vi "Main.vi"() -> ()   [LabVIEW 2017, in "Vibratome.lvlib"]
uses:
  Vibratome.lvlib
  Controls/Down.ctl
  Controls/Up.ctl
  Drivers/ASI/Public/Utility/Axis Name.ctl
  Support VIs/Message Queue/Enqueue Message (Single).vi
  Support VIs/Message Queue/Enqueue Message (Multiple).vi
  Support VIs/Stop Event/Stop Event.lvlib
  Support VIs/Message Queue/Message Queue.lvlib
  Piezo Controller/Piezo Controller.lvlib
  Stage/Stage.lvlib
  Drivers/ASI/ASI TG-1000.lvlib
panel:
  in  "Specimen X":cluster{"X-":T1, "X+":T2}
  in  "Set X Pos":T3
  in  "Abort":bool
  in  "Run":bool
  in  "Specimen Z":cluster{"Z-":T1, "Z+":T2}
  in  "Blade":cluster{"F-":T1, "F+":T2}
  in  "Oscillator Settings":cluster{"Amplitude":dbl, "Frequency":dbl}={"Amplitude"=5.0, "Frequency"=40.0} {"Frequency" format="%.0f Hz"; "Amplitude" format="%.0f V"}
  in  "Speed":dbl min=0.0 step=0.1 format="%.1f mm/s"
  in  "Thickness":dbl=50.0 min=0.0 max=10000.0 step=1.0 format="%.0f um"
  # "Blade"
  # "Specimen"
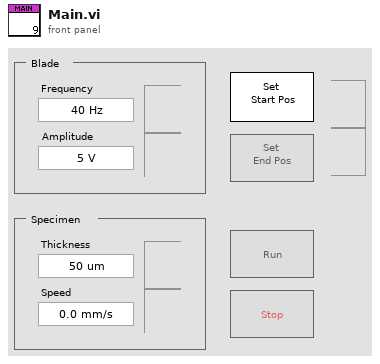
[diagram p1: front panel]
types:
  T1 = typedef "Vibratome.lvlib/Down.ctl" = bool
  T2 = typedef "Vibratome.lvlib/Up.ctl" = bool
  T3 = cluster{"Set Start Pos":bool, "Set End Pos":bool}
  T4 = typedef "Vibratome.lvlib/Message Queues.ctl" = cluster{"UI Message":refnum<queue>, "Piezo Message":refnum<queue>, "Stage Message":refnum<queue>}
  T5 = typedef "Drivers.lvlib/ASI TG-1000.lvlib/Axis Name.ctl" = enum8{"undefined", "A", "B", "C", "D", "E", "F", "G", "H", "I", "J", "K", "L", "M", "N", "O", "P", "Q", "R", "S", "T", "U", "V", "W", "X", "Y", "Z"}
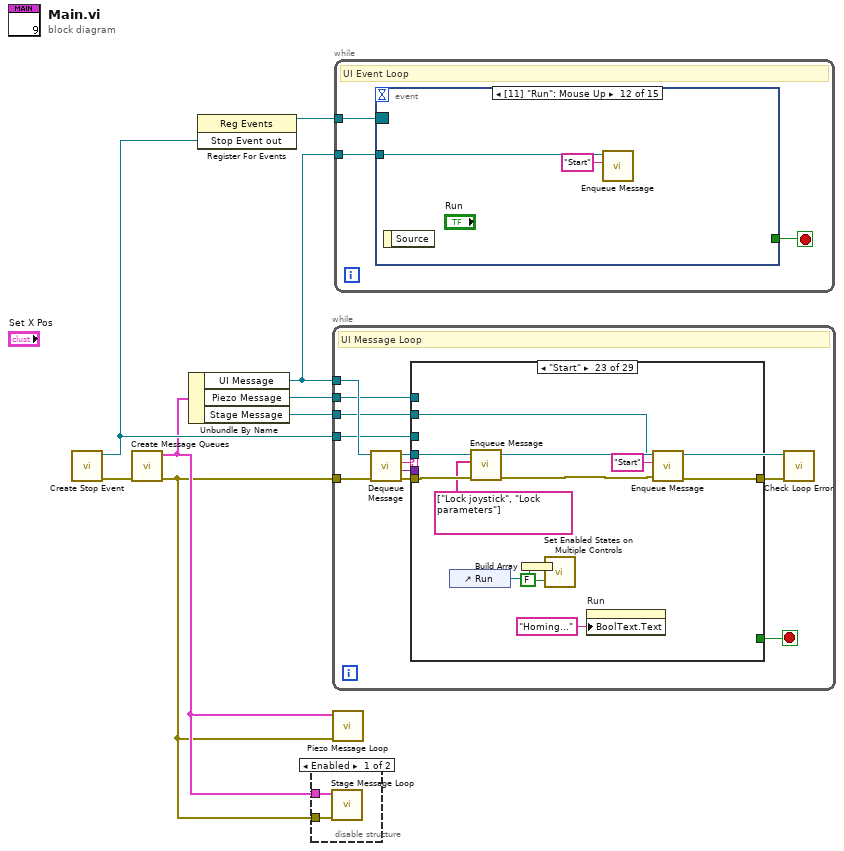
[diagram p0: block diagram]
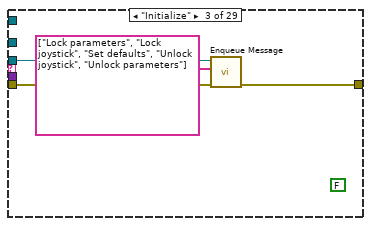
[diagram p5: hidden frame]
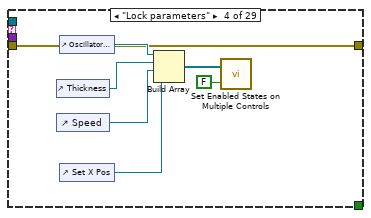
[diagram p6: hidden frame]
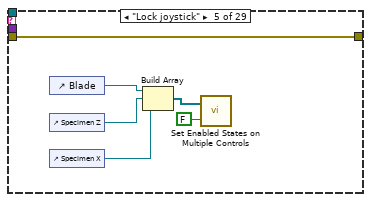
[diagram p7: hidden frame]
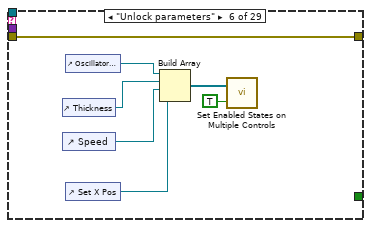
[diagram p8: hidden frame]
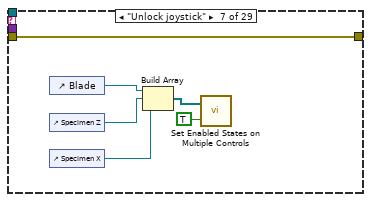
[diagram p9: hidden frame]
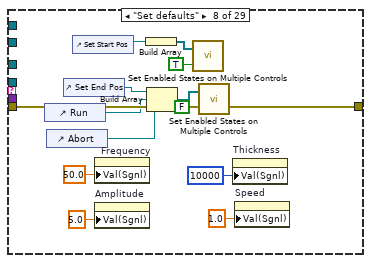
[diagram p10: hidden frame]
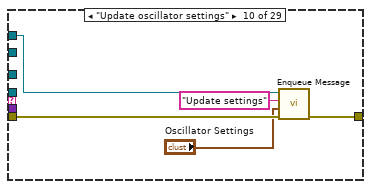
[diagram p12: hidden frame]
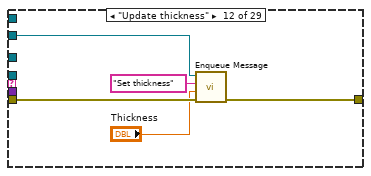
[diagram p14: hidden frame]
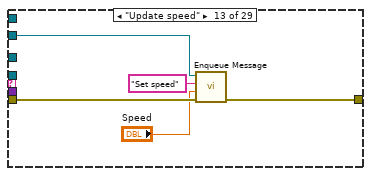
[diagram p15: hidden frame]
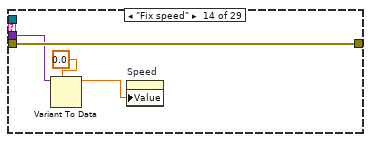
[diagram p16: hidden frame]
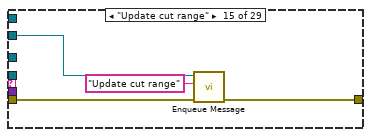
[diagram p17: hidden frame]
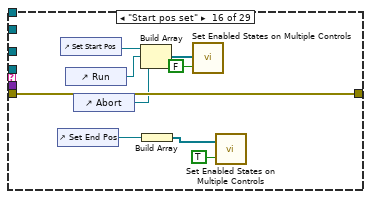
[diagram p18: hidden frame]
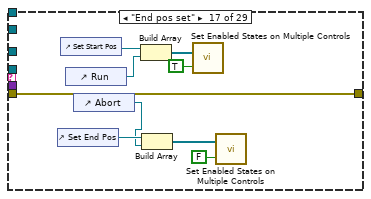
[diagram p19: hidden frame]
diagram:
  n1 = call "Create Stop Event.vi"() -> ("error out"=w8:errorcluster, "Stop Event out"=w3:refnum<user-event>)  [unwired: 10 in]
  n2 = call "Create Message Queues.vi"("error in (no error)"=w8) -> ("error out"=w1:errorcluster, "Message Queues"=w2:T4)  [unwired: 9 in]
  n3 = Unbundle By Name(w2) -> ("UI Message"=w6:refnum<queue>, "Piezo Message"=w5:refnum<queue>, "Stage Message"=w4:refnum<queue>)
  n4 = register-events(w3) -> (reference out=w7:refnum<event-registration>)  [unwired: 2 in, 1 out]
  n5 = disable-structure shown="Enabled" {
    disable-tunnel: w2 -> [w10 _]
    disable-tunnel: w1 -> [w9 _]
    frame Enabled {
      n6 = call "Stage Message Loop.vi"("error in (no error)"=w9, "Message Queues"=w10) -> ()  [unwired: 9 in, 1 out]
    }
    frame Disabled {
    }
  }
  n7 = while {
    tunnel: w6 -> [w21]
    tunnel: w1 -> [w20]
    tunnel: w5 -> [w13]
    tunnel: w4 -> [w12]
    tunnel: w3 -> [w14]
    stop <- w15 stop-if-true
    # "UI Message Loop"
    n8 = call "Dequeue Message.vi"("error in (no error)"=w20, "Message Queue in"=w21) -> ("error out"=w18:errorcluster, "Data"=w11:variant, "State"=w19:string, "Message Queue out"=w17:refnum<queue>)  [unwired: 6 in]
    n9 = case shown="\"Start\"" w19 {
      tunnel: w17 -> [_ _ w27 _ _ _ _ _ _ _ _ _ _ _ _ _ _ _ _ _ _ _ w155 _ _ w184 _ _ _]
      tunnel: w18 -> [w22 w23 w26 w28 w35 w41 w48 w62 w67 w72 w73 w78 w83 w87 w91 w100 w109 w110 w122 w134 w146 w147 w156 w160 w176 w180 w190 w191 w198]
      tunnel: [w22 w23 w25 w28 w35 w41 w48 w62 w67 w71 w73 w77 w82 w87 w88 w100 w109 w110 w118 w130 w142 w147 w158 w159 w172 w185 w190 w191 w201] -> w16
      tunnel: [_ _ _ _ _ _ _ _ _ _ _ _ _ _ _ _ _ _ _ _ _ _ _ _ _ _ _ _ TRUE] -> w15
      tunnel: w14 -> [_ _ _ _ _ _ _ _ _ _ _ _ _ _ _ _ _ _ _ _ _ _ _ _ _ _ _ _ w200]
      tunnel: w13 -> [_ _ _ _ _ _ _ _ _ w70 _ _ _ _ _ _ _ _ _ _ _ _ _ w161 _ w178 _ _ w196]
      tunnel: w12 -> [_ _ _ _ _ _ _ _ _ _ _ w76 w81 _ w90 _ _ _ w121 w133 w145 _ w157 _ w175 _ _ _ w195]
      tunnel: w11 -> [_ _ _ _ _ _ _ _ _ _ _ _ _ w86 _ _ _ _ w111 w123 w135 _ _ _ _ _ _ _ _]
      frame Default {
      }
      frame "--- SETUP ---" {
      }
      frame "Initialize" {
        (unwired) FALSE ("Running?")
        n10 = call-poly "Enqueue Message.vi"("error in (no error)"=w26, "States"=string[] ["Lock parameters", "Lock joystick", "Set defaults", "Unlock joystick", "Unlock parameters"], "Message Queue in"=w27) -> ("error out"=w25:errorcluster)  [unwired: 7 in, 1 out]
      }
      frame "Lock parameters" {
        n11 = control-ref of="Thickness"() -> (w33:refnum<vi>)
        n12 = control-ref of="Speed"() -> (w32:refnum<vi>)
        n13 = control-ref of="Oscillator Settings"() -> (w34:refnum<vi>)
        n14 = control-ref of="Set X Pos"() -> (w31:refnum<vi>)
        n15 = Build Array(w34, w33, w32, w31) -> (w30:refnum<vi>[])
        n16 = call "Set Enabled States on Multiple Controls.vi"("Enable?"=FALSE, "Control Refnums"=w30) -> ()  [unwired: 1 in]
      }
      frame "Lock joystick" {
        n17 = control-ref of="Blade"() -> (w40:refnum<vi>)
        n18 = control-ref of="Specimen Z"() -> (w39:refnum<vi>)
        n19 = control-ref of="Specimen X"() -> (w38:refnum<vi>)
        n20 = Build Array(w40, w39, w38) -> (w37:refnum<vi>[])
        n21 = call "Set Enabled States on Multiple Controls.vi"("Enable?"=FALSE, "Control Refnums"=w37) -> ()  [unwired: 1 in]
      }
      frame "Unlock parameters" {
        n22 = control-ref of="Thickness"() -> (w46:refnum<vi>)
        n23 = control-ref of="Speed"() -> (w45:refnum<vi>)
        n24 = control-ref of="Oscillator Settings"() -> (w47:refnum<vi>)
        n25 = control-ref of="Set X Pos"() -> (w44:refnum<vi>)
        n26 = Build Array(w47, w46, w45, w44) -> (w43:refnum<vi>[])
        n27 = call "Set Enabled States on Multiple Controls.vi"("Enable?"=TRUE, "Control Refnums"=w43) -> ()  [unwired: 1 in]
      }
      frame "Unlock joystick" {
        n28 = control-ref of="Blade"() -> (w53:refnum<vi>)
        n29 = control-ref of="Specimen Z"() -> (w52:refnum<vi>)
        n30 = control-ref of="Specimen X"() -> (w51:refnum<vi>)
        n31 = Build Array(w53, w52, w51) -> (w50:refnum<vi>[])
        n32 = call "Set Enabled States on Multiple Controls.vi"("Enable?"=TRUE, "Control Refnums"=w50) -> ()  [unwired: 1 in]
      }
      frame "Set defaults" {
        n33 = control-ref of="Run"() -> (w55:refnum<vi>)
        n34 = control-ref of="Abort"() -> (w54:refnum<vi>)
        n35 = control-ref of="Set End Pos"() -> (w58:refnum<vi>)
        n36 = control-ref of="Set Start Pos"() -> (w61:refnum<vi>)
        n37 = property on="Frequency" class="DigNum (strict)"("Val(Sgnl)"=50.0 ("Value (Signaling)")) -> ()  [unwired: 2 in, 2 out]
        n38 = property on="Amplitude" class="DigNum (strict)"("Val(Sgnl)"=5.0 ("Value (Signaling)")) -> ()  [unwired: 2 in, 2 out]
        n39 = Build Array(w61) -> (w60:refnum<vi>[])
        n40 = Build Array(w58, w55, w54) -> (w57:refnum<vi>[])
        n41 = call "Set Enabled States on Multiple Controls.vi"("Enable?"=TRUE, "Control Refnums"=w60) -> ()  [unwired: 1 in]
        n42 = call "Set Enabled States on Multiple Controls.vi"("Enable?"=FALSE, "Control Refnums"=w57) -> ()  [unwired: 1 in]
        n43 = property on="Thickness" class="DigNum (strict)"("Val(Sgnl)"=10000 ("Value (Signaling)")) -> ()  [unwired: 2 in, 2 out]
        n44 = property on="Speed" class="DigNum (strict)"("Val(Sgnl)"=1.0 ("Value (Signaling)")) -> ()  [unwired: 2 in, 2 out]
      }
      frame "--- PIEZO ---" {
      }
      frame "Update oscillator settings" {
        n45 = call-poly "Enqueue Message.vi"("error in (no error)"=w72, "Data"="Oscillator Settings", "State"="Update settings", "Message Queue in"=w70) -> ("error out"=w71:errorcluster)  [unwired: 6 in, 1 out]
      }
      frame "--- STAGE ---" {
      }
      frame "Update thickness" {
        n46 = call-poly "Enqueue Message.vi"("error in (no error)"=w78, "Data"="Thickness", "State"="Set thickness", "Message Queue in"=w76) -> ("error out"=w77:errorcluster)  [unwired: 6 in, 1 out]
      }
      frame "Update speed" {
        n47 = call-poly "Enqueue Message.vi"("error in (no error)"=w83, "Data"="Speed", "State"="Set speed", "Message Queue in"=w81) -> ("error out"=w82:errorcluster)  [unwired: 6 in, 1 out]
      }
      frame "Fix speed" {
        n48 = Variant To Data(type=0.0, Variant=w86) -> (data=w85:dbl)  [unwired: 1 in, 1 out]
        n49 = property on="Speed" class="DigNum (strict)"("Value"=w85) -> ()  [unwired: 2 in, 2 out]
      }
      frame "Update cut range" {
        n50 = call-poly "Enqueue Message.vi"("error in (no error)"=w91, "State"="Update cut range", "Message Queue in"=w90) -> ("error out"=w88:errorcluster)  [unwired: 7 in, 1 out]
      }
      frame "Start pos set" {
        n51 = control-ref of="Set End Pos"() -> (w96:refnum<vi>)
        n52 = control-ref of="Set Start Pos"() -> (w99:refnum<vi>)
        n53 = control-ref of="Run"() -> (w95:refnum<vi>)
        n54 = control-ref of="Abort"() -> (w94:refnum<vi>)
        n55 = Build Array(w99, w95, w94) -> (w98:refnum<vi>[])
        n56 = Build Array(w96) -> (w93:refnum<vi>[])
        n57 = call "Set Enabled States on Multiple Controls.vi"("Enable?"=FALSE, "Control Refnums"=w98) -> ()  [unwired: 1 in]
        n58 = call "Set Enabled States on Multiple Controls.vi"("Enable?"=TRUE, "Control Refnums"=w93) -> ()  [unwired: 1 in]
      }
      frame "End pos set" {
        n59 = control-ref of="Set End Pos"() -> (w105:refnum<vi>)
        n60 = control-ref of="Set Start Pos"() -> (w108:refnum<vi>)
        n61 = control-ref of="Run"() -> (w104:refnum<vi>)
        n62 = control-ref of="Abort"() -> (w101:refnum<vi>)
        n63 = Build Array(w108, w104) -> (w107:refnum<vi>[])
        n64 = Build Array(w105, w101) -> (w103:refnum<vi>[])
        n65 = call "Set Enabled States on Multiple Controls.vi"("Enable?"=TRUE, "Control Refnums"=w107) -> ()  [unwired: 1 in]
        n66 = call "Set Enabled States on Multiple Controls.vi"("Enable?"=FALSE, "Control Refnums"=w103) -> ()  [unwired: 1 in]
      }
      frame "--- JOG ---" {
      }
      frame "Jog X" {
        n67 = call-poly "Enqueue Message.vi"("error in (no error)"=w122, "Data"=Axis_Name."X" ("active axis"), "State"="Select axis", "Message Queue in"=w121) -> ("error out"=w116:errorcluster, "Message Queue out"=w115:refnum<queue>)  [unwired: 6 in]
        n68 = call-poly "Enqueue Message.vi"("error in (no error)"=w116, "Data"=w111, "State"="Set jog direction", "Message Queue in"=w115) -> ("error out"=w113:errorcluster, "Message Queue out"=w114:refnum<queue>)  [unwired: 6 in]
        n69 = call-poly "Enqueue Message.vi"("error in (no error)"=w113, "State"="Jogging", "Message Queue in"=w114) -> ("error out"=w118:errorcluster)  [unwired: 7 in, 1 out]
      }
      frame "Jog Z" {
        n70 = call-poly "Enqueue Message.vi"("error in (no error)"=w134, "Data"=Axis_Name."Z" ("active axis"), "State"="Select axis", "Message Queue in"=w133) -> ("error out"=w128:errorcluster, "Message Queue out"=w127:refnum<queue>)  [unwired: 6 in]
        n71 = call-poly "Enqueue Message.vi"("error in (no error)"=w128, "Data"=w123, "State"="Set jog direction", "Message Queue in"=w127) -> ("error out"=w125:errorcluster, "Message Queue out"=w126:refnum<queue>)  [unwired: 6 in]
        n72 = call-poly "Enqueue Message.vi"("error in (no error)"=w125, "State"="Jogging", "Message Queue in"=w126) -> ("error out"=w130:errorcluster)  [unwired: 7 in, 1 out]
      }
      frame "Jog F" {
        n73 = call-poly "Enqueue Message.vi"("error in (no error)"=w146, "Data"=Axis_Name."F" ("active axis"), "State"="Select axis", "Message Queue in"=w145) -> ("error out"=w140:errorcluster, "Message Queue out"=w139:refnum<queue>)  [unwired: 6 in]
        n74 = call-poly "Enqueue Message.vi"("error in (no error)"=w140, "Data"=w135, "State"="Set jog direction", "Message Queue in"=w139) -> ("error out"=w137:errorcluster, "Message Queue out"=w138:refnum<queue>)  [unwired: 6 in]
        n75 = call-poly "Enqueue Message.vi"("error in (no error)"=w137, "State"="Jogging", "Message Queue in"=w138) -> ("error out"=w142:errorcluster)  [unwired: 7 in, 1 out]
      }
      frame "--- OPS ---" {
      }
      frame "Start" {
        n76 = control-ref of="Run"() -> (w150:refnum<vi>)
        n77 = call-poly "Enqueue Message.vi"("error in (no error)"=w156, "States"=string[] ["Lock joystick", "Lock parameters"], "Message Queue in"=w155) -> ("error out"=w148:errorcluster)  [unwired: 7 in, 1 out]
        n78 = Build Array(w150) -> (w152:refnum<vi>[])
        n79 = call "Set Enabled States on Multiple Controls.vi"("Enable?"=FALSE, "Control Refnums"=w152) -> ()  [unwired: 1 in]
        n80 = property on="Run" class="Bool (strict)"("BoolText.Text"="Homing..." ("Boolean Text.Text")) -> ()  [unwired: 2 in, 2 out]
        n81 = call-poly "Enqueue Message.vi"("error in (no error)"=w148, "State"="Start", "Message Queue in"=w157) -> ("error out"=w158:errorcluster)  [unwired: 7 in, 1 out]
      }
      frame "Started" {
        n82 = control-ref of="Abort"() -> (w164:refnum<vi>)
        n83 = Build Array(w164) -> (w166:refnum<vi>[])
        n84 = property on="Run" class="Bool (strict)"("BoolText.Text"="Running" ("Boolean Text.Text")) -> ()  [unwired: 2 in, 2 out]
        n85 = call "Set Enabled States on Multiple Controls.vi"("Enable?"=TRUE, "Control Refnums"=w166) -> ()  [unwired: 1 in]
        n86 = call-poly "Enqueue Message.vi"("error in (no error)"=w160, "State"="Start", "Message Queue in"=w161) -> ("error out"=w159:errorcluster)  [unwired: 7 in, 1 out]
      }
      frame "Stop" {
        n87 = control-ref of="Abort"() -> (w169:refnum<vi>)
        n88 = property on="Run" class="Bool (strict)"("BoolText.Text"="Run" ("Boolean Text.Text")) -> ()  [unwired: 2 in, 2 out]
        n89 = Build Array(w169) -> (w171:refnum<vi>[])
        n90 = call-poly "Enqueue Message.vi"("High Priority?"=TRUE, "error in (no error)"=w176, "State"="Stop", "Message Queue in"=w175) -> ("error out"=w172:errorcluster)  [unwired: 6 in, 1 out]
        n91 = property on="Abort" class="Bool (strict)"("BoolText.Text"="Stopping..." ("Boolean Text.Text")) -> ()  [unwired: 2 in, 2 out]
        n92 = call "Set Enabled States on Multiple Controls.vi"("Enable?"=FALSE, "Control Refnums"=w171) -> ()  [unwired: 1 in]
      }
      frame "Stopped" {
        n93 = control-ref of="Run"() -> (w186:refnum<vi>)
        n94 = control-ref of="Set X Pos"() -> (w189:refnum<vi>)
        n95 = call-poly "Enqueue Message.vi"("High Priority?"=TRUE, "error in (no error)"=w180, "State"="Stop", "Message Queue in"=w178) -> ("error out"=w179:errorcluster)  [unwired: 6 in, 1 out]
        n96 = Build Array(w189, w186) -> (w188:refnum<vi>[])
        n97 = call "Set Enabled States on Multiple Controls.vi"("Enable?"=TRUE, "Control Refnums"=w188) -> ()  [unwired: 1 in]
        n98 = property on="Abort" class="Bool (strict)"("BoolText.Text"="Stop" ("Boolean Text.Text")) -> ()  [unwired: 2 in, 2 out]
        n99 = call-poly "Enqueue Message.vi"("error in (no error)"=w179, "States"=string[] ["Unlock parameters", "Unlock joystick"], "Message Queue in"=w184) -> ("error out"=w185:errorcluster)  [unwired: 7 in, 1 out]
      }
      frame "--- MISC ---" {
      }
      frame "Error" {
      }
      frame "Exit" {
        w194 = "Exit" ("State")
        n100 = call-poly "Enqueue Message.vi"("High Priority?"=TRUE, "error in (no error)"=w198, "State"=w194, "Message Queue in"=w196) -> ("error out"=w199:errorcluster)  [unwired: 6 in, 1 out]
        n101 = call-poly "Enqueue Message.vi"("High Priority?"=TRUE, "error in (no error)"=w199, "State"=w194, "Message Queue in"=w195) -> ("error out"=w197:errorcluster)  [unwired: 6 in, 1 out]
        n102 = call "Fire Stop Event.vi"("error in (no error)"=w197, "Stop Event in"=w200) -> ("error out"=w201:errorcluster)  [unwired: 8 in, 1 out]
      }
    }
    n103 = call "Check Loop Error.vi"("error in (no error)"=w16, "Message Queue in"=w17) -> ()  [unwired: 7 in, 3 out]
  }
  n104 = call "Piezo Message Loop.vi"("error in (no error)"=w1, "Message Queues"=w2) -> ()  [unwired: 9 in, 1 out]
  n105 = while {
    tunnel: w7 -> [w205]
    tunnel: w6 -> [w203]
    stop <- w204 stop-if-true
    # "UI Event Loop"
    n106 = event shown="[11] \"Run\": Mouse Up" {
      selector: w205 -> [_ _ _ _ _ _ _ _ _ _ _ _ _ _ _]
      dyn-events: _ -> [_ _ _ _ _ _ _ _ _ _ _ _ _ _ _]
      timeout: _ -> [_ _ _ _ _ _ _ _ _ _ _ _ _ _ _]
      tunnel: [_ _ _ _ _ _ _ _ _ _ _ _ _ _ TRUE] -> w204
      tunnel: w203 -> [w208 w211 w214 w217 w220 w223 w225 w227 w229 w231 w233 w235 w237 w240 _]
      event Mouse Down {
        n107 = event-data() -> ()  [unwired: 1 in, 2 out]
        n108 = call-poly "Enqueue Message.vi"("Data"=TRUE, "State"="Jog X", "Message Queue in"=w208) -> ()  [unwired: 7 in, 2 out]
      }
      event Mouse Down {
        n109 = event-data() -> ()  [unwired: 1 in, 2 out]
        n110 = call-poly "Enqueue Message.vi"("Data"=FALSE, "State"="Jog X", "Message Queue in"=w211) -> ()  [unwired: 7 in, 2 out]
      }
      event Mouse Down {
        n111 = event-data() -> ()  [unwired: 1 in, 2 out]
        n112 = call-poly "Enqueue Message.vi"("Data"=TRUE, "State"="Jog Z", "Message Queue in"=w214) -> ()  [unwired: 7 in, 2 out]
      }
      event Mouse Down {
        n113 = event-data() -> ()  [unwired: 1 in, 2 out]
        n114 = call-poly "Enqueue Message.vi"("Data"=FALSE, "State"="Jog Z", "Message Queue in"=w217) -> ()  [unwired: 7 in, 2 out]
      }
      event Mouse Down {
        n115 = event-data() -> ()  [unwired: 1 in, 2 out]
        n116 = call-poly "Enqueue Message.vi"("Data"=TRUE, "State"="Jog F", "Message Queue in"=w220) -> ()  [unwired: 7 in, 2 out]
      }
      event Mouse Down {
        n117 = event-data() -> ()  [unwired: 1 in, 2 out]
        n118 = call-poly "Enqueue Message.vi"("Data"=FALSE, "State"="Jog F", "Message Queue in"=w223) -> ()  [unwired: 7 in, 2 out]
      }
      event "Specimen X", "Specimen Z", "Blade": Mouse Up {
        n119 = event-data() -> ()  [unwired: 1 in, 1 out]
        n120 = call-poly "Enqueue Message.vi"("State"="Stop", "Message Queue in"=w225) -> ()  [unwired: 8 in, 2 out]
      }
      event "Oscillator Settings": Value Change {
        n121 = event-data() -> ()  [unwired: 1 in, 1 out]
        n122 = call-poly "Enqueue Message.vi"("State"="Update oscillator settings", "Message Queue in"=w227) -> ()  [unwired: 8 in, 2 out]
      }
      event "Thickness": Value Change {
        n123 = event-data() -> ()  [unwired: 1 in, 1 out]
        n124 = call-poly "Enqueue Message.vi"("State"="Update thickness", "Message Queue in"=w229) -> ()  [unwired: 8 in, 2 out]
      }
      event "Speed": Value Change {
        n125 = event-data() -> ()  [unwired: 1 in, 1 out]
        n126 = call-poly "Enqueue Message.vi"("State"="Update speed", "Message Queue in"=w231) -> ()  [unwired: 8 in, 2 out]
      }
      event "Set X Pos": Mouse Up {
        n127 = event-data() -> ()  [unwired: 1 in, 1 out]
        n128 = call-poly "Enqueue Message.vi"("State"="Update cut range", "Message Queue in"=w233) -> ()  [unwired: 8 in, 2 out]
      }
      event "Run": Mouse Up {
        n129 = event-data() -> ()  [unwired: 1 in, 1 out]
        n130 = call-poly "Enqueue Message.vi"("State"="Start", "Message Queue in"=w235) -> ()  [unwired: 8 in, 2 out]
      }
      event "Abort": Mouse Up {
        n131 = event-data() -> ()  [unwired: 1 in, 1 out]
        n132 = call-poly "Enqueue Message.vi"("State"="Stop", "Message Queue in"=w237) -> ()  [unwired: 8 in, 2 out]
      }
      event Application Instance Close {
        n133 = event-data() -> ()  [unwired: 1 in, 1 out]
        n134 = call-poly "Enqueue Message.vi"("High Priority?"=TRUE, "State"="Exit", "Message Queue in"=w240) -> ()  [unwired: 7 in, 2 out]
      }
      event User Event {
        n135 = event-data() -> ()  [unwired: 1 in, 1 out]
      }
    }
  }
